vi "PXI-Get Output Terminal Configuration.vi"(7 "term config in":i32(ring)=-1 items=["Default"=-1, "RSE"=10083, "Differential"=10106, "Pseudodifferential"=12529], 11 "error in (no error)":errorcluster, 13 "key":string) -> (8 "term config out":i32(ring)=-1 items=["Default"=-1, "RSE"=10083, "Differential"=10106, "Pseudodifferential"=12529], 15 "error out":errorcluster)   [LabVIEW 2020]
uses:
  <vilib>/Utility/config.llb/Read Key (String).vi
  <vilib>/Utility/config.llb/NI_LVConfig.lvlib
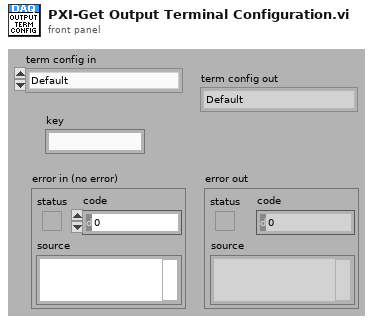
[diagram p1: front panel]
types:
  T1 = typedef "LVStringsAndValuesArrayTypeDef_I32.ctl" = cluster{"String":string, "Value":i32}[]
  T2 = typedef "NI_LVConfig.lvlib/Config Data RefNum.ctl" = refnum<k1>
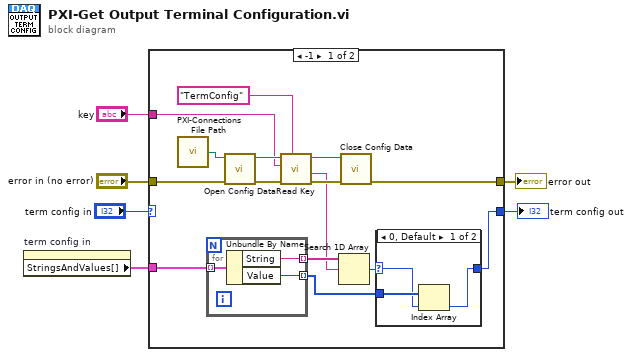
[diagram p0: block diagram]
diagram:
  n1 = property on="term config in" class="Ring (strict)"() -> ("StringsAndValues[]"=w2:T1)  [unwired: 2 in, 2 out]
  n2 = case shown="-1" "term config in" {
    selector: "term config in" -> [_ w29]
    tunnel: "error in (no error)" -> [w21 w30]
    tunnel: [w15 w30] -> w5
    tunnel: "key" -> [w13 _]
    tunnel: w2 -> [w9 _]
    tunnel: [w7 w29] -> w1
    frame -1 {
      n3 = call "PXI-Connections File Path.vi"() -> ("Path"=w14:path)  [unwired: 1 in]
      n4 = for {
        tunnel: w9 -> [w28] mode=indexing
        tunnel: [w27] -> w12 mode=indexing
        tunnel: [w26] -> w10 mode=indexing
        n5 = Unbundle By Name(w28) -> ("String"=w27:string, "Value"=w26:i32)
      }
      n6 = call <vilib>:"Open Config Data.vi"("error in (no error)"=w21, "configuration file path"=w14) -> ("error out"=w20:errorcluster, "refnum"=w19:T2)  [unwired: 7 in, 1 out]
      n7 = call-poly <vilib>:"Read Key.vi"("section"="TermConfig", "error in (no error)"=w20, "key"=w13, "refnum"=w19) -> ("error out"=w17:errorcluster, "value"=w8:string, "refnum out"=w16:T2)  [unwired: 4 in, 1 out]
      n8 = Search 1D Array(1D array=w12, element=w8) -> (index of element=w11:i32)  [unwired: 1 in]
      n9 = call <vilib>:"Close Config Data.vi"("error in (no error)"=w17, "refnum"=w16) -> ("error out"=w15:errorcluster)  [unwired: 8 in, 1 out]
      n10 = case shown="0, Default" w11 {
        selector: w11 -> [w23 w25]
        tunnel: [w22 w25] -> w7
        tunnel: w10 -> [w24 _]
        frame 0, Default {
          n11 = Index Array(array=w24, index=w23) -> (element=w22:i32)
        }
        frame -1 {
        }
      }
    }
    frame 1, Default {
    }
  }
  "error out" <- w5
  "term config out" <- w1
